vi "Build Vizualization Filter.vi"(11 "Filters":T1[](array[typedef])) -> (3 "Filter out":refnum<class "Filter.lvclass">)   [LabVIEW 2016, in "RM.Server.lvlib"]
uses:
  RM.Server.lvlib
  Client/Test CD/FPGA RM Test Client/Source/System Explorer/Filters/NOT Filter/NOT Filter.lvclass
  Client/Test CD/FPGA RM Test Client/Source/System Explorer/Filters/And Filter/AND Filter.lvclass
  Client/Test CD/FPGA RM Test Client/Source/System Explorer/Filters/OR Filter/OR Filter.lvclass
  Client/Test CD/FPGA RM Test Client/Source/System Explorer/Filters/Filter Parent/Filter.lvclass
  viz_filter.ctl
  viz_filter options.ctl
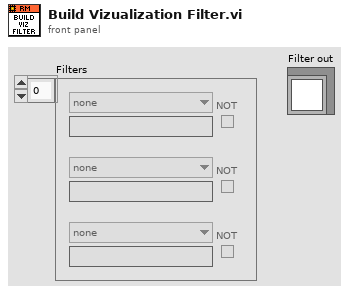
[diagram p1: front panel]
types:
  T1 = typedef "RM.Server.lvlib/viz_filter options.ctl" = cluster{"Filter Options":cluster{"Filter Type":T2, "Filter Value":string, "NOT":bool}}
  T2 = typedef "RM.Server.lvlib/viz_filter.ctl" = enum16{"none", "RIO Device", "Resource Name", "Input Type", "Datatype"}
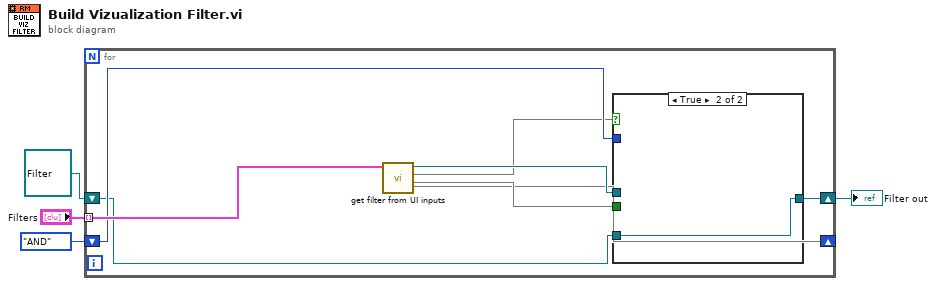
[diagram p0: block diagram]
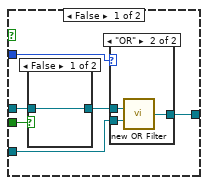
[diagram p2: hidden frame]
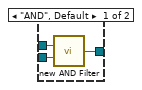
[diagram p3: hidden frame]
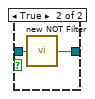
[diagram p4: hidden frame]
diagram:
  n1 = for {
    tunnel: "Filters" -> [w12] mode=indexing
    shift-right: [w6] -> w4
    shift-left: refnum<class "Filter.lvclass"> refnum ("Filter.lvclass") -> [w7]
    shift-right: [w9] -> _
    shift-left: enum16{"AND", "OR"}."AND" ("next filter boolean") -> [w8]
    n2 = call "get filter from UI inputs.vi"("Filter Type"=w12) -> (1:w11, 2:w5, "Filter out"=w10:refnum<class "Filter.lvclass">, 4:w9)  [unwired: 7 in]
    n3 = case shown="True" w5 {
      tunnel: w11 -> [w18 _]
      tunnel: w10 -> [w17 _]
      tunnel: w8 -> [w16 _]
      tunnel: w7 -> [w14 w28]
      tunnel: [w13 w28] -> w6
      frame False {
        n4 = case shown="False" w18 {
          tunnel: w17 -> [w25 w27]
          tunnel: [w25 w26] -> w15
          frame False {
          }
          frame True {
            n5 = call "new NOT Filter.vi"("a"=w27) -> ("not a"=w26:refnum<class "Filter.lvclass">)  [unwired: 14 in]
          }
        }
        n6 = case shown="\"OR\"" w16 {
          tunnel: w15 -> [w21 w24]
          tunnel: w14 -> [w20 w23]
          tunnel: [w19 w22] -> w13
          frame "AND", Default {
            n7 = call "new AND Filter.vi"("a"=w21, "b"=w20) -> ("a and b"=w19:refnum<class "Filter.lvclass">)  [unwired: 13 in]
          }
          frame "OR" {
            n8 = call "new OR Filter.vi"("a"=w24, "b"=w23) -> ("a or b"=w22:refnum<class "Filter.lvclass">)  [unwired: 13 in]
          }
        }
      }
      frame True {
      }
    }
  }
  "Filter out" <- w4
